vi "KB-循环滤波.vi"() -> ()   [LabVIEW 2015]
panel:
  out "数组 2":dbl[](array[numeric])
  out "外环波形图 3":dbl[](graph)
  out "数组":dbl[](array[numeric])
  out "外环波形图 2":dynamicdata(graph)
  in  "外环波形图":dbl[](graph)
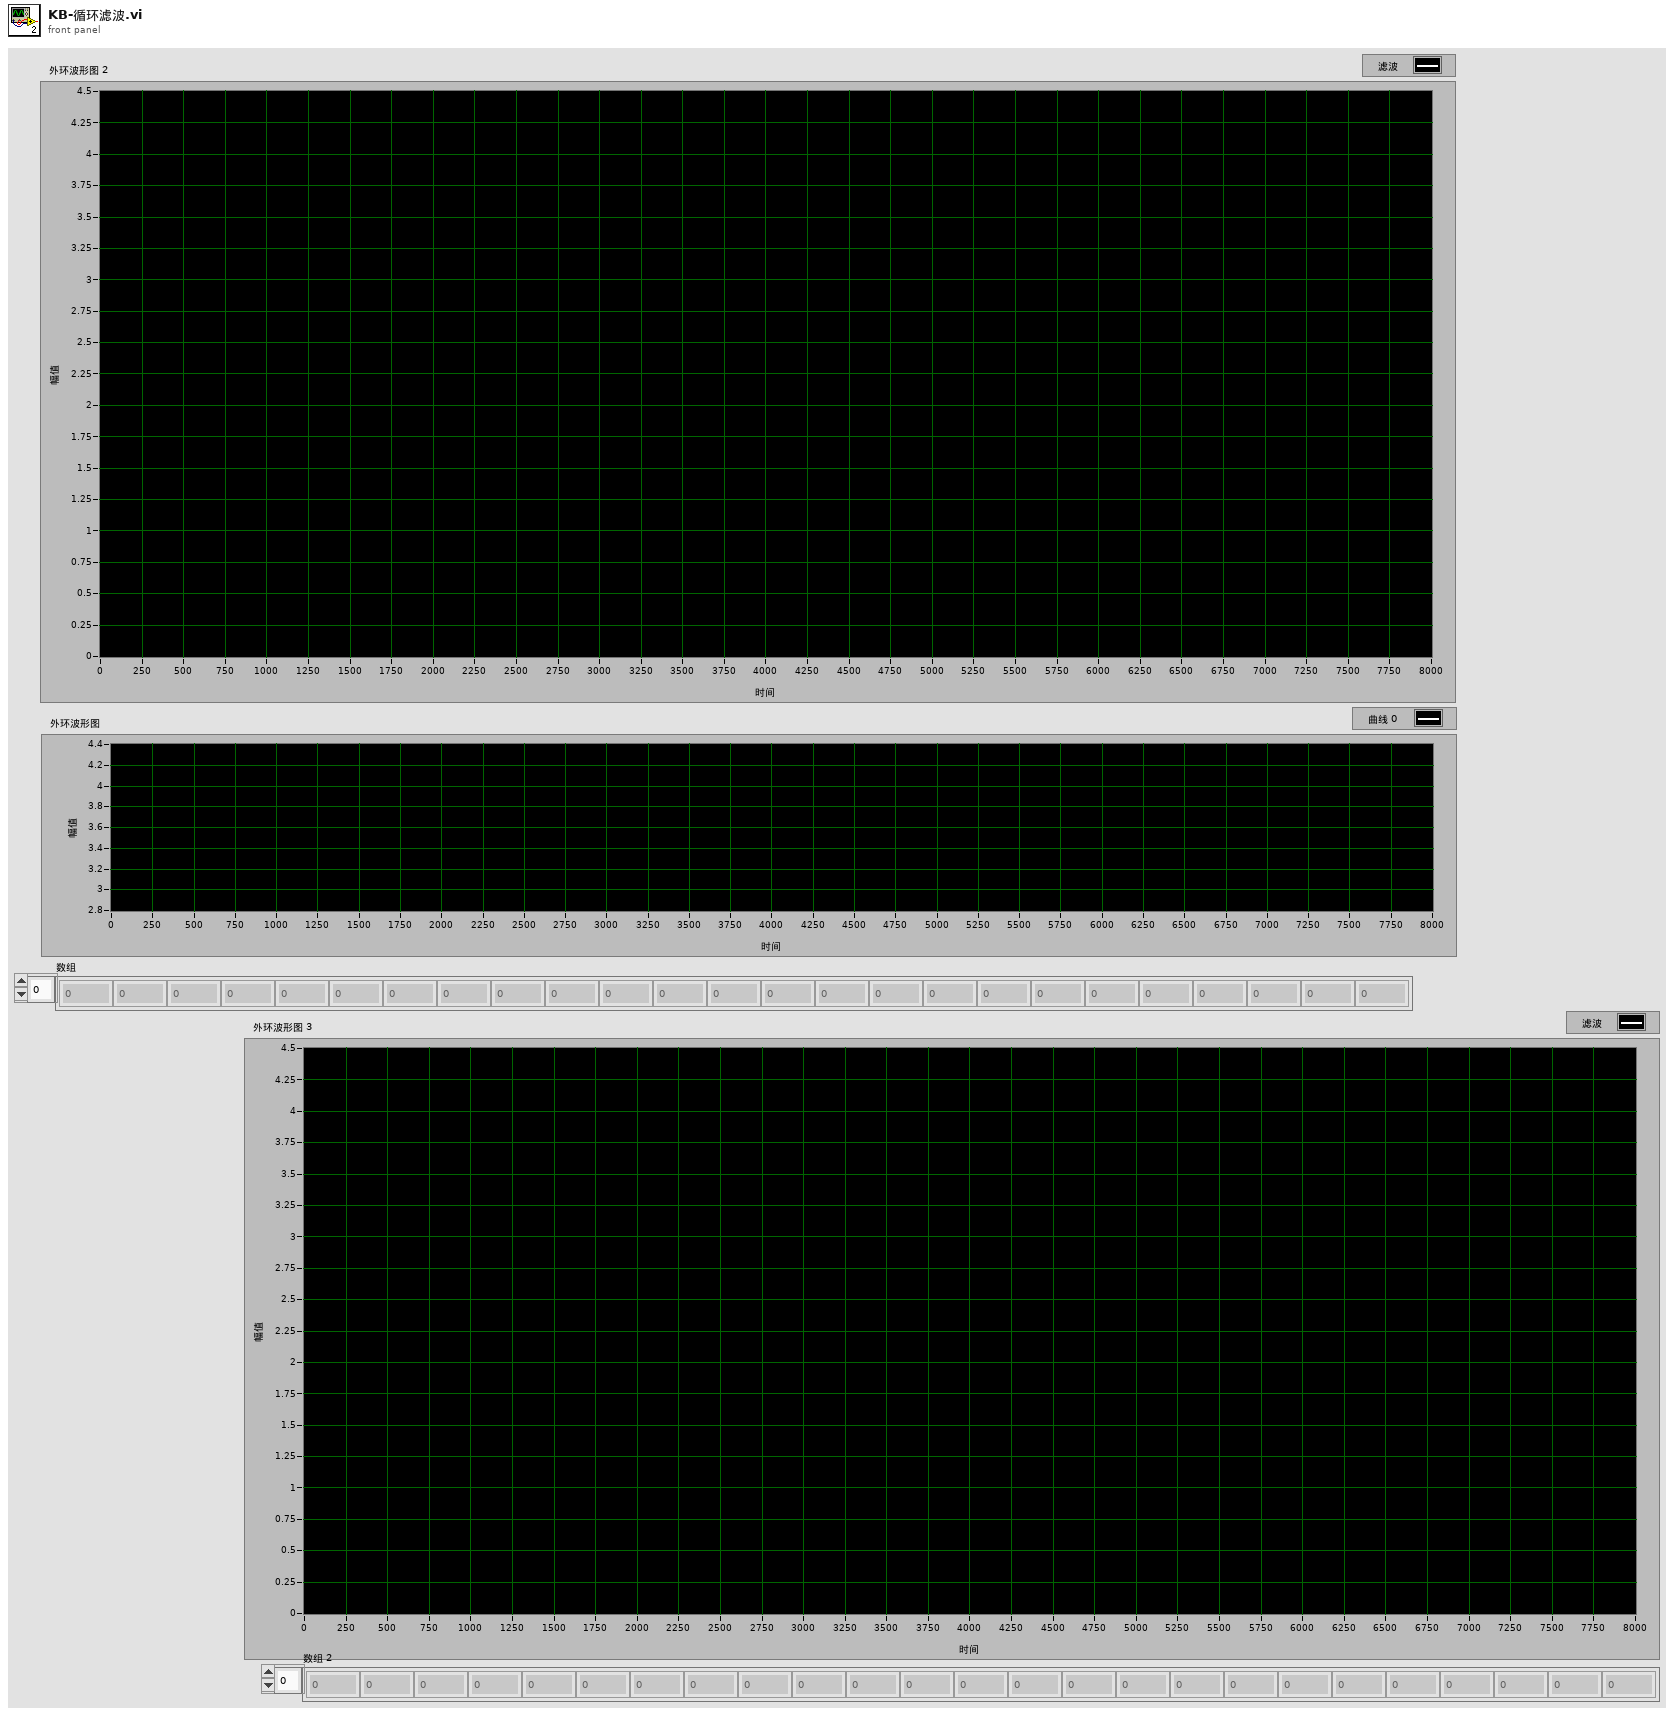
[diagram p1: front panel]
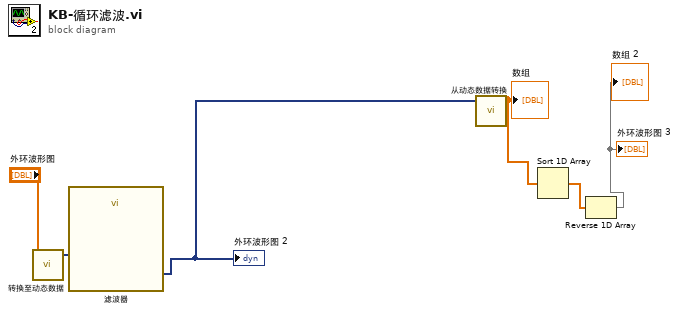
[diagram p0: block diagram]
diagram:
  n1 = call "转换至动态数据"("Array"="外环波形图") -> ("Dynamic Data Type"=w5:dynamicdata)  [unwired: 3 in]
  n2 = call "滤波器"("Signal"=w5) -> ("Filtered Signal"=w4:dynamicdata)  [unwired: 9 in, 1 out]
  "外环波形图 2" <- w4
  n3 = call "从动态数据转换"("Dynamic Data Type"=w4) -> ("Array"=w3:dbl[])  [unwired: 3 in]
  "数组" <- w3
  n4 = Sort 1D Array(array=w3) -> (sorted array=w2:dbl[])
  n5 = Reverse 1D Array(array=w2) -> (reversed array=→"外环波形图 3" →"数组 2":dbl[])
